vi "Test Verify throws Error if No Expectations Configured.vi"(8 "error in (no error)":errorcluster, 11 "Expectation Test In":refnum<class "Expectation Test.lvclass">) -> (0 "error out":errorcluster, 3 "Expectation Test Out":refnum<class "Expectation Test.lvclass">)   [LabVIEW 2020, in "Expectation Test.lvclass"]
uses:
  Expectation Test.lvclass
  C:/Program Files (x86)/National Instruments/LabVIEW 2020/vi.lib/Astemes/LUnit/Test Case.lvclass
  <vilib>/Astemes/LUnit/Test Case.lvclass/Test Case.ctl
  <vilib>/Astemes/LUnit/Append Fail Result.vi
  <vilib>/Astemes/LUnit/Append Pass Result.vi
  Expectation Test.lvclass/Expectation Test.ctl
  <vilib>/Astemes/LUnit/Test Case.lvclass
  source/Framework/Verifier/Verifier.lvclass
  Test Doubles/Test Interface Responsive Mock/Test Interface Mock.lvclass
  C:/git/astemes-lmock/source/Framework/Mock/LMock Mock.lvclass
  C:/git/astemes-lmock/tests/Test Doubles/Test Interface Responsive Mock/Test Interface Mock.lvclass
  C:/git/astemes-lmock/tests/Test Doubles/Test Interface/Test Interface.lvclass
  C:/Program Files (x86)/National Instruments/LabVIEW 2020/vi.lib/Astemes/LUnit/LUnit Runnable.lvclass
  C:/git/astemes-lmock/tests/Expectation Test/Expectation Test.lvclass
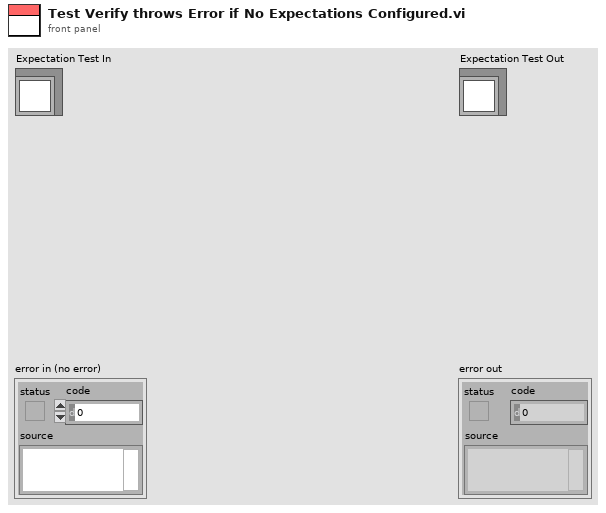
[diagram p1: front panel]
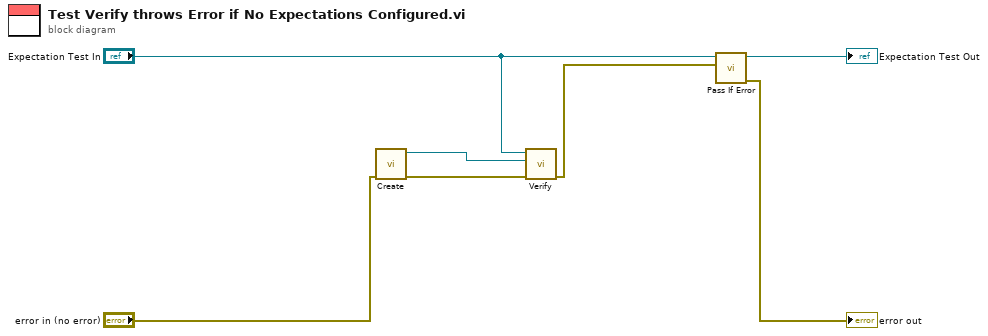
[diagram p0: block diagram]
diagram:
  n1 = call "Create.vi"("error in (no error)"="error in (no error)") -> ("error out"=w2:errorcluster, "Test Interface Mock Out"=w3:refnum<class "Test Interface Mock.lvclass">)  [unwired: 9 in]
  n2 = call "Verify.vi"("error in (no error)"=w2, "Mock"=w3, "LUnit Test Case In"="Expectation Test In") -> ("error out"=w4:errorcluster)  [unwired: 7 in, 1 out]
  n3 = call <vilib>:"Pass If Error.vi"("Assert error"=w4, "LUnit Test Case In"="Expectation Test In") -> ("error out"=→"error out":errorcluster, "LUnit Test Case Out"=→"Expectation Test Out":refnum<class "Expectation Test.lvclass">)  [unwired: 8 in]
